vi "GetAScanDataHdr.vi"(8 "错误输入（无错误）":errorcluster, 10 "采样深度":i32, 11 "需要获取的通道":u8) -> (0 "错误输出":errorcluster, 1 "Data":dbl[](array[numeric]), 2 "Time":dbl[](array[numeric]), 3 "波形数据":dbl[][](array[numeric]))   [LabVIEW 2018]
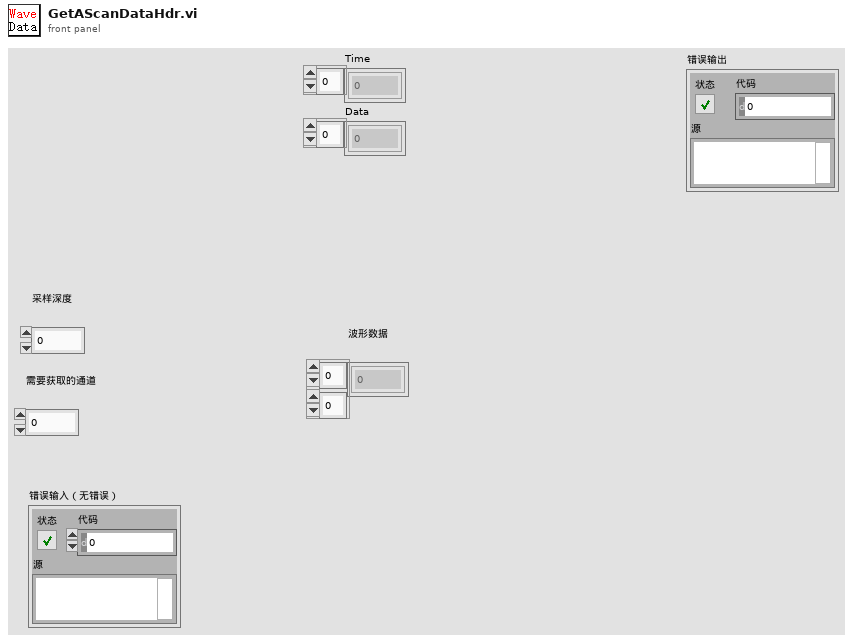
[diagram p1: front panel]
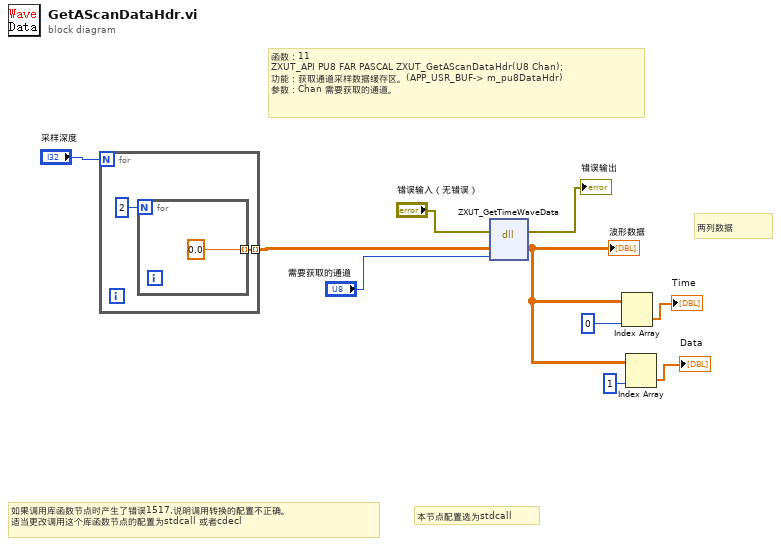
[diagram p0: block diagram]
diagram:
  # "两列数据"
  # "本节点配置选为stdcall"
  # "如果调用库函数节点时产生了错误1517,说明调用转换的配置不正确。\n适当更改调用这个库函数节点的配置为stdcall 或者cdecl"
  # "函数：11\nZXUT_API PU8\tFAR PASCAL ZXUT_GetAScanDataHdr(U8 Chan);\n功能：获取通道采样数据缓存区。(APP_USR_BUF-> m_pu8DataHdr)\n参数：Chan 需要获取的通道。"
  n1 = for {
    N: "采样深度" -> [_]
    tunnel: [w11] -> w9 mode=indexing
    n2 = for {
      N: 2 -> [_]
      tunnel: [0.0] -> w11 mode=indexing
    }
  }
  n3 = dll-call lib="PTH2Rabs E软件项目超声超声子VI函数VI\tTCG处理ZXUTConfigMgr.dll" fn="ZXUT_GetTimeWaveData"(error in="错误输入（无错误）", "buff"=w9, "Chan"="需要获取的通道") -> (error out=→"错误输出":errorcluster, "buff"=w1:dbl[][])  [unwired: 4 in, 1 out]
  "波形数据" <- w1
  n4 = Index Array(array=w1, index (col)=0 ("索引 (行)")) -> (element=→"Time":dbl[])  [unwired: 1 in]
  n5 = Index Array(array=w1, index (col)=1 ("禁用的索引 (列)")) -> (element=→"Data":dbl[])  [unwired: 1 in]
